vi "Selection Template.vi"() -> ()   [LabVIEW 2014]
panel:
  out "Current State":string
  in  "Recycling Conainer?":bool
  in  "Totes Collected":i8(knob) scale=0.0..3.0
  in  "Direction?":bool
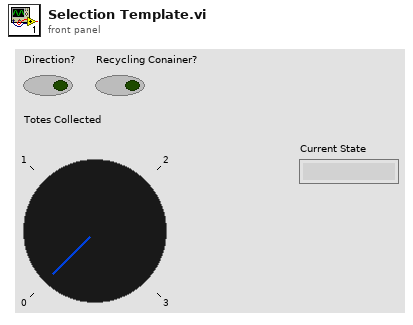
[diagram p1: front panel]
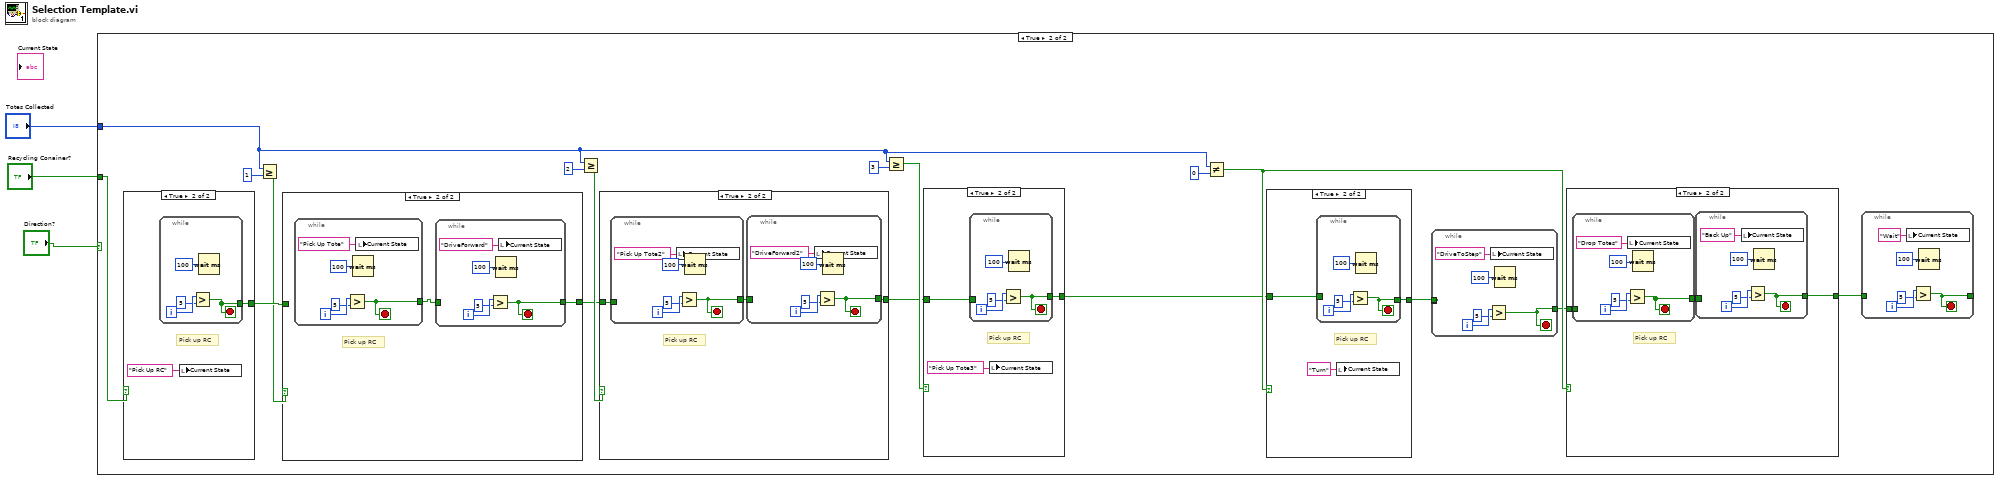
[diagram p0: block diagram]
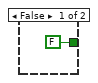
[diagram p3: hidden frame]
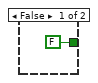
[diagram p4: hidden frame]
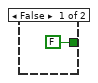
[diagram p5: hidden frame]
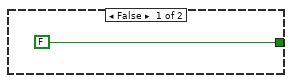
[diagram p6: hidden frame]
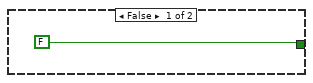
[diagram p7: hidden frame]
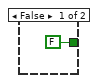
[diagram p8: hidden frame]
diagram:
  n1 = case shown="True" "Direction?" {
    tunnel: "Totes Collected" -> [_ w12]
    tunnel: "Recycling Conainer?" -> [_ w20]
    frame False {
    }
    frame True {
      n2 = case shown="True" w20 {
        tunnel: [FALSE w90] -> w19
        frame False {
        }
        frame True {
          # "Pick up RC"
          n3 = while {
            tunnel: [w92] -> w90
            i -> [w94]
            stop <- w92 stop-if-true
            n4 = Greater?(x=w94, y=5) -> (0:w92:bool)
            n5 = Wait (ms)(milliseconds to wait=u32 100) -> ()  [unwired: 1 out]
          }
          n6 = local write "Current State"("Pick Up RC" ("Current State")) -> ()
        }
      }
      n7 = Greater Or Equal?(x=w12, y=i8 1) -> (x >= y?=w17:bool)
      n8 = case shown="True" w17 {
        tunnel: w19 -> [_ _]
        tunnel: [FALSE w77] -> w7
        frame False {
        }
        frame True {
          # "Pick up RC"
          n9 = while {
            tunnel: [w85] -> w78
            i -> [w87]
            stop <- w85 stop-if-true
            n10 = Greater?(x=w87, y=5) -> (0:w85:bool)
            n11 = Wait (ms)(milliseconds to wait=u32 100) -> ()  [unwired: 1 out]
            n12 = local write "Current State"("Pick Up Tote" ("Current State")) -> ()
          }
          n13 = while {
            tunnel: [w80] -> w77
            tunnel: w78 -> [_]
            i -> [w82]
            stop <- w80 stop-if-true
            n14 = Greater?(x=w82, y=5) -> (0:w80:bool)
            n15 = Wait (ms)(milliseconds to wait=u32 100) -> ()  [unwired: 1 out]
            n16 = local write "Current State"("DriveForward" ("Current State")) -> ()
          }
        }
      }
      n17 = Greater Or Equal?(x=w12, y=i8 2) -> (x >= y?=w15:bool)
      n18 = case shown="True" w15 {
        tunnel: [FALSE w63] -> w6
        tunnel: w7 -> [_ w65]
        frame False {
        }
        frame True {
          # "Pick up RC"
          n19 = while {
            tunnel: [w72] -> w64
            tunnel: w65 -> [_]
            i -> [w74]
            stop <- w72 stop-if-true
            n20 = local write "Current State"("Pick Up Tote2" ("Current State")) -> ()
            n21 = Greater?(x=w74, y=5) -> (0:w72:bool)
            n22 = Wait (ms)(milliseconds to wait=u32 100) -> ()  [unwired: 1 out]
          }
          n23 = while {
            tunnel: [w67] -> w63
            tunnel: w64 -> [_]
            i -> [w69]
            stop <- w67 stop-if-true
            n24 = local write "Current State"("DriveForward2" ("Current State")) -> ()
            n25 = Greater?(x=w69, y=5) -> (0:w67:bool)
            n26 = Wait (ms)(milliseconds to wait=u32 100) -> ()  [unwired: 1 out]
          }
        }
      }
      n27 = Greater Or Equal?(x=w12, y=i8 3) -> (x >= y?=w13:bool)
      n28 = case shown="True" w13 {
        tunnel: [FALSE w56] -> w8
        tunnel: w6 -> [_ w55]
        frame False {
        }
        frame True {
          # "Pick up RC"
          n29 = while {
            tunnel: [w58] -> w56
            tunnel: w55 -> [_]
            i -> [w60]
            stop <- w58 stop-if-true
            n30 = Greater?(x=w60, y=5) -> (0:w58:bool)
            n31 = Wait (ms)(milliseconds to wait=u32 100) -> ()  [unwired: 1 out]
          }
          n32 = local write "Current State"("Pick Up Tote3" ("Current State")) -> ()
        }
      }
      n33 = Not Equal?(x=w12, y=i8 0) -> (x != y?=w9:bool)
      n34 = case shown="True" w9 {
        tunnel: [FALSE w48] -> w10
        tunnel: w8 -> [_ w47]
        frame False {
        }
        frame True {
          # "Pick up RC"
          n35 = while {
            tunnel: [w51] -> w48
            tunnel: w47 -> [_]
            i -> [w53]
            stop <- w51 stop-if-true
            n36 = Greater?(x=w53, y=5) -> (0:w51:bool)
            n37 = Wait (ms)(milliseconds to wait=u32 100) -> ()  [unwired: 1 out]
          }
          n38 = local write "Current State"("Turn" ("Current State")) -> ()
        }
      }
      n39 = while {
        tunnel: [w41] -> _
        tunnel: w10 -> [w41]
        tunnel: [w40] -> w5
        i -> [w44]
        stop <- w40 stop-if-true
        n40 = Greater?(x=w44, y=5) -> (0:w40:bool)
        n41 = local write "Current State"("DriveToStep" ("Current State")) -> ()
        n42 = Wait (ms)(milliseconds to wait=u32 100) -> ()  [unwired: 1 out]
      }
      n43 = case shown="True" w9 {
        tunnel: w5 -> [_ w29]
        tunnel: [FALSE w27] -> w4
        frame False {
        }
        frame True {
          # "Pick up RC"
          n44 = while {
            tunnel: [w36] -> w28
            tunnel: w29 -> [_]
            i -> [w38]
            stop <- w36 stop-if-true
            n45 = Greater?(x=w38, y=5) -> (0:w36:bool)
            n46 = local write "Current State"("Drop Totes" ("Current State")) -> ()
            n47 = Wait (ms)(milliseconds to wait=u32 100) -> ()  [unwired: 1 out]
          }
          n48 = while {
            tunnel: [w31] -> w27
            tunnel: w28 -> [_]
            i -> [w33]
            stop <- w31 stop-if-true
            n49 = local write "Current State"("Back Up" ("Current State")) -> ()
            n50 = Greater?(x=w33, y=5) -> (0:w31:bool)
            n51 = Wait (ms)(milliseconds to wait=u32 100) -> ()  [unwired: 1 out]
          }
        }
      }
      n52 = while {
        tunnel: [w22] -> _
        tunnel: w4 -> [_]
        i -> [w24]
        stop <- w22 stop-if-true
        n53 = local write "Current State"("Wait" ("Current State")) -> ()
        n54 = Greater?(x=w24, y=5) -> (0:w22:bool)
        n55 = Wait (ms)(milliseconds to wait=u32 100) -> ()  [unwired: 1 out]
      }
    }
  }
